vi "Coloration.vi"(8 "String":string, 9 "Code":refnum<vi>, 11 "Front Panel":refnum<vi>) -> ()   [LabVIEW 2019]
panel:
  out "Value":string
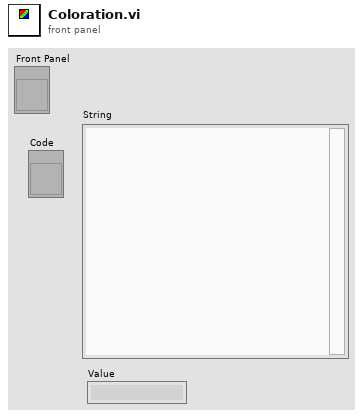
[diagram p1: front panel]
types:
  T1 = typedef "LVSelectionTypeDef.ctl" = cluster{"Selection Start":u32, "Selection End":u32}
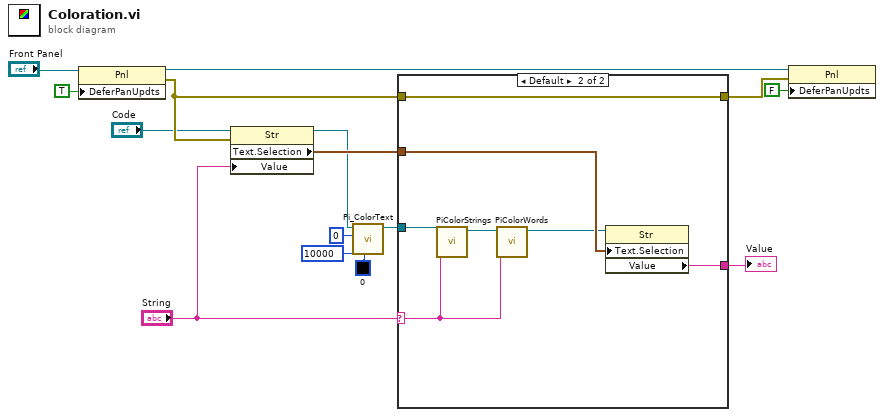
[diagram p0: block diagram]
diagram:
  n1 = property class="Pnl"(reference="Front Panel", "DeferPanUpdts"=TRUE ("Defer Panel Updates")) -> (reference out=w13:refnum<vi>, error out=w11:errorcluster)  [unwired: 1 in]
  n2 = property on="Property Node" class="Str"(reference="Code", error in=w11, "Value"="String") -> (reference out=w6:refnum<vi>, "Text.Selection"=w15:T1)  [unwired: 1 out]
  n3 = call "Pi_ColorText.vi"("Color"=u32 0, "End"=10000, "Start"=0, "String in"=w6) -> ("String out"=w7:refnum<vi>)  [unwired: 7 in]
  n4 = case shown="Default" "String" {
    selector: "String" -> [w16 w19]
    tunnel: w7 -> [_ w21]
    tunnel: w15 -> [_ w22]
    tunnel: [w16 w23] -> w14
    tunnel: [w17 w24] -> w12
    tunnel: w11 -> [w17 w24]
    frame "" {
    }
    frame Default {
      n5 = call "PiColorStrings.vi"("String"=w19, "String in"=w21) -> ("String out"=w20:refnum<vi>)  [unwired: 9 in]
      n6 = call "PiColorWords.vi"("String"=w19, "String in"=w20) -> ("String out"=w18:refnum<vi>)  [unwired: 9 in]
      n7 = property on="Property Node" class="Str"(reference=w18, "Text.Selection"=w22) -> ("Value"=w23:string)  [unwired: 1 in, 2 out]
    }
  }
  "Value" <- w14
  n8 = property class="Pnl"(reference=w13, error in=w12, "DeferPanUpdts"=FALSE ("Defer Panel Updates")) -> ()  [unwired: 2 out]
